vi "Exchange_Subtracks_Statuses-1.vi"(5 "[IN] Statuses wit\nhout prehistory":i16[](array[numeric]), 6 "[IN] Row index \nProblem Point":i32, 7 "[IN] Statuses\nwith problem":i16[](array[numeric])) -> (1 "[OUT] Reconnected statuses\n(posthistory after deleted \ncrossconnected point)":i16[](array[numeric]), 3 "[OUT] Reconnected statuses\nPrehistory + alternative prob\nlem point":i16[](array[numeric]))   [LabVIEW 2017]
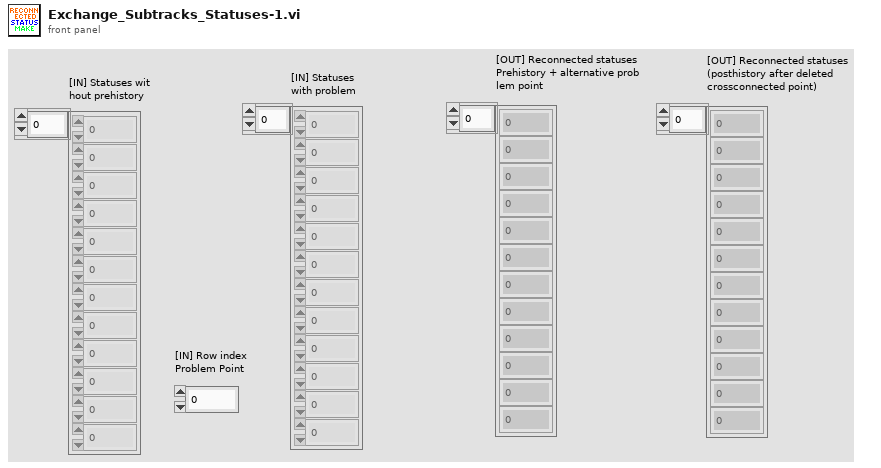
[diagram p1: front panel]
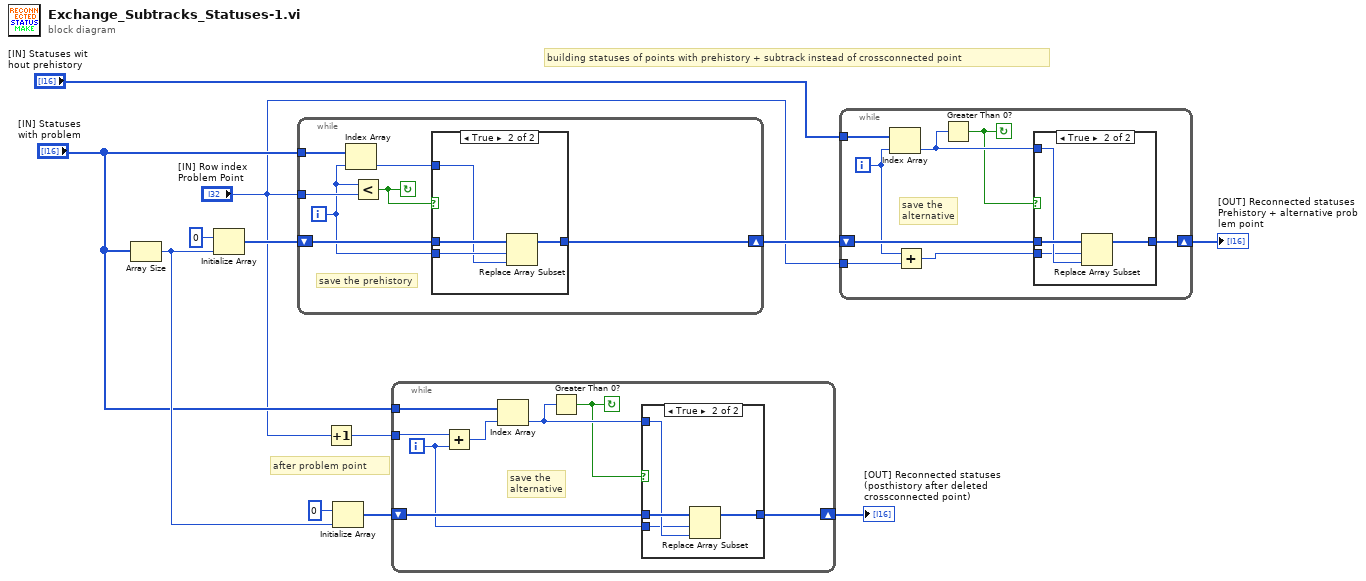
[diagram p0: block diagram]
diagram:
  # "after problem point"
  # "building statuses of points with prehistory + subtrack instead of crossconnected point"
  n1 = Array Size(array="[IN] Statuses\nwith problem") -> (size(s)=w10:i32)
  n2 = Initialize Array(i16 0 ("element"), w10) -> (w9:i16[])
  n3 = while {
    shift-right: [w16] -> w8
    shift-left: w9 -> [w17]
    tunnel: "[IN] Statuses\nwith problem" -> [w15]
    tunnel: "[IN] Row index \nProblem Point" -> [w19]
    i -> [w14]
    stop <- w18 continue-if-true
    # "save the prehistory"
    n4 = Index Array(array=w15, index=w14) -> (element=w13:i16)
    n5 = Less?(x=w14, y=w19) -> (x < y?=w18:bool)
    n6 = case shown="True" w18 {
      tunnel: w17 -> [w20 w24]
      tunnel: w14 -> [_ w23]
      tunnel: [w20 w21] -> w16
      tunnel: w13 -> [_ w22]
      frame False {
      }
      frame True {
        n7 = Replace Array Subset(array=w24, new element=w22, index=w23) -> (w21:i16[])
      }
    }
  }
  n8 = Increment(x="[IN] Row index \nProblem Point") -> (x+1=w1:i32)
  n9 = Initialize Array(i16 0 ("element"), w10) -> (w5:i16[])
  n10 = while {
    shift-right: [w31] -> w4
    shift-left: w5 -> [w32]
    tunnel: "[IN] Statuses\nwith problem" -> [w30]
    tunnel: w1 -> [w27]
    i -> [w26]
    stop <- w28 continue-if-true
    # "save the \nalternative"
    n11 = Add(x=w27, y=w26) -> (x+y=w25:i32)
    n12 = Index Array(array=w30, index=w25) -> (element=w29:i16)
    n13 = Greater Than 0?(x=w29) -> (x > 0?=w28:bool)
    n14 = case shown="True" w28 {
      tunnel: w29 -> [_ w36]
      tunnel: w32 -> [w33 w37]
      tunnel: w26 -> [_ w35]
      tunnel: [w33 w34] -> w31
      frame False {
      }
      frame True {
        n15 = Replace Array Subset(array=w37, new element=w36, index=w35) -> (w34:i16[])
      }
    }
  }
  "[OUT] Reconnected statuses\n(posthistory after deleted \ncrossconnected point)" <- w4
  n16 = while {
    shift-right: [w44] -> w6
    shift-left: w8 -> [w45]
    tunnel: "[IN] Statuses wit\nhout prehistory" -> [w42]
    tunnel: "[IN] Row index \nProblem Point" -> [w43]
    i -> [w41]
    stop <- w39 continue-if-true
    # "save the \nalternative"
    n17 = Index Array(array=w42, index=w41) -> (element=w40:i16)
    n18 = Add(x=w41, y=w43) -> (x+y=w38:i32)
    n19 = Greater Than 0?(x=w40) -> (x > 0?=w39:bool)
    n20 = case shown="True" w39 {
      tunnel: w40 -> [_ w49]
      tunnel: w45 -> [w46 w50]
      tunnel: w38 -> [_ w48]
      tunnel: [w46 w47] -> w44
      frame False {
      }
      frame True {
        n21 = Replace Array Subset(array=w50, new element=w49, index=w48) -> (w47:i16[])
      }
    }
  }
  "[OUT] Reconnected statuses\nPrehistory + alternative prob\nlem point" <- w6
